vi "GT Set Dac.vi"(7 "count":i16, 8 "error in (no error)":errorcluster caption="错误输入（无错误）", 9 "pValue":i16[](array[numeric]), 10 "dac":i16, 11 "cardNum":i16) -> (0 "error out":errorcluster caption="错误输出", 1 "pValue out":i16[](array[numeric]), 3 "function return":i16)   [LabVIEW 2020, in "gts.lvlib"]
doc: "GT_API GT_SetDac(short cardNum,short dac,short *pValue,short count=1);"
uses:
  gts.lvlib
  dll/32bit/multi_card/gts.dll
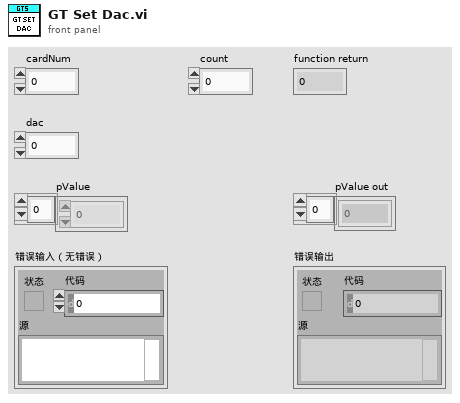
[diagram p1: front panel]
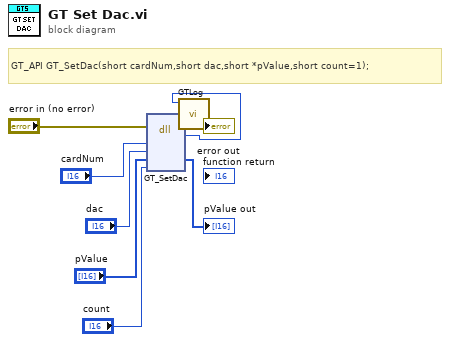
[diagram p0: block diagram]
diagram:
  # "GT_API GT_SetDac(short cardNum,short dac,short *pValue,short count=1);"
  n1 = dll-call lib="C:/1228/dll/32bit/multi_card/gts.dll" fn="GT_SetDac"(error in="error in (no error)", "cardNum"="cardNum", "dac"="dac", "pValue"="pValue", "count"="count") -> (error out=w3:errorcluster, "返回类型"=w1:i16, "pValue"=→"pValue out":i16[])  [unwired: 5 in, 1 out]
  n2 = call "GTLog.vi"("error in (no error)"=w3, "Numeric"=w1) -> ("error out"=→"error out":errorcluster)  [unwired: 9 in]
